vi "Shutdown Core.vi"(8 "error in (no error)":errorcluster, 11 "NI-SWITCH Consumer in":refnum<class "%DEVICE% Consumer.lvclass">) -> (0 "error out":errorcluster, 3 "NI-SWITCH Consumer out":refnum<class "%DEVICE% Consumer.lvclass">)   [LabVIEW 2017, in "%DEVICE% Messaging.lvlib" / "%DEVICE% Consumer.lvclass"]
uses:
  %DEVICE% Consumer.lvclass
  %DEVICE% Consumer.lvclass/%DEVICE% Consumer.ctl
  Session Type.ctl
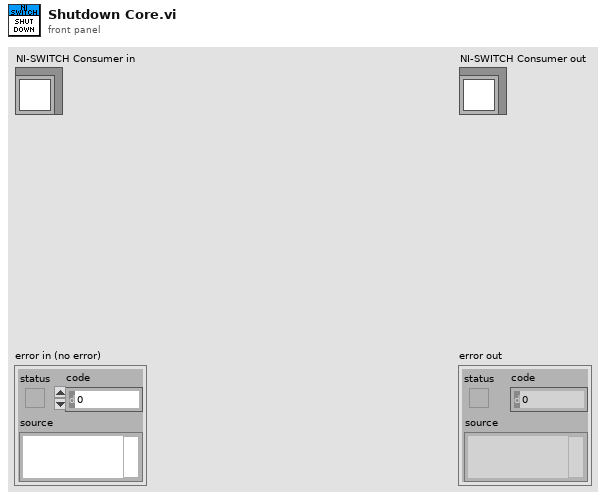
[diagram p1: front panel]
types:
  T1 = typedef "%DEVICE% Messaging.lvlib/%DEVICE% Consumer.lvclass/Session Type.ctl" = picture
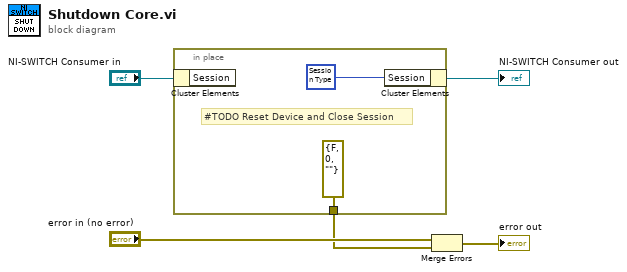
[diagram p0: block diagram]
diagram:
  n1 = in-place {
    in-place-border: [errorcluster {"status"=FALSE, "code"=0, "source"=""} ("error out")] -> w3
    # "#TODO Reset Device and Close Session"
    n2 = in-place-cluster #1("NI-SWITCH Consumer in") -> ()  [unwired: 1 out]
    n3 = in-place-cluster #1("Session"=T1 data[5B]) -> (→"NI-SWITCH Consumer out":refnum<class "%DEVICE% Consumer.lvclass">)
  }
  n4 = Merge Errors("error in (no error)", w3) -> (→"error out":errorcluster)
